vi "ReadAODVolume.vi"(8 "error in":errorcluster, 11 "FilePath":path) -> (0 "error out":errorcluster, 3 "settings_um":dbl[][](array[numeric]))   [LabVIEW 2014]
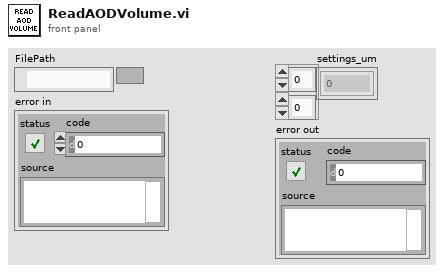
[diagram p1: front panel]
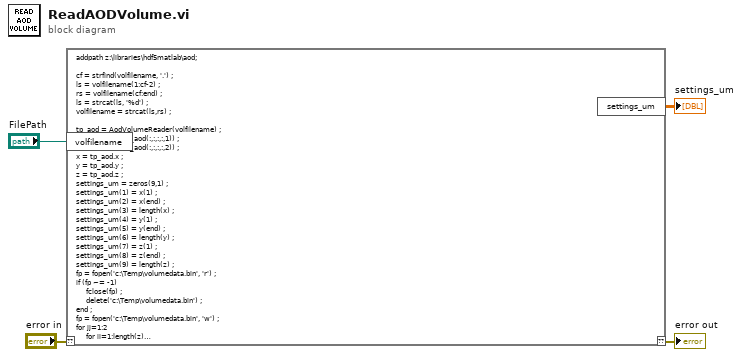
[diagram p0: block diagram]
diagram:
  n1 = script code="addpath z:\\libraries\\hdf5matlab\\aod;\n\ncf = strfind(volfilename, '.') ;\nls = volfilename(1:cf-2) ;\nrs = volfilename(cf:end) ;\nls = strcat(ls, '%d') ;\nvolfilename = strcat(ls,rs) ;\n\ntp_aod = AodVolumeReader(volfilename) ;\nvc1 = double(tp_aod(:,:,:,:,1)) ;\nvc2 = double(tp_aod(:,:,:,:,2)) ;\nx = tp_aod.x ;\ny = tp_aod.y ;\nz = tp_aod.z ;\nsettings_um = zeros(9,1) ;\nsettings_um(1) = x(1) ;\nsettings_um(2) = x(end) ;\nsettings_um(3) = length(x) ;\nsettings_um(4) = y(1) ;\nsettings_um(5) = y(end) ;\nsettings_um(6) = length(y) ;\nsettings_um(7) = z(1) ;\nsettings_um(8) = z(end) ;\nsettings_um(9) = length(z) ;\nfp = fopen('c:\\Temp\\volumedata.bin', 'r') ;\nif (fp ~= -1)\n     fclose(fp) ;\n     delete('c:\\Temp\\volumedata.bin') ;\nend ;\nfp = fopen('c:\\Temp\\volumedata.bin', 'w') ;\nfor jj=1:2\n     for ii=1:length(z)\n          if (jj==1)\n             tvol = vc1(:,:,ii) ; % write each frame in row order\n          else\n             tvol = vc2(:,:,ii) ;\n          end ;\n          fwrite(fp, tvol, 'int32') ;\n     end ;\nend ;\nfclose(fp) ;\nclearvars vc1 vc2 tvol"("??"="error in", "volfilename"="FilePath") -> ("??"=→"error out":errorcluster, "settings_um"=→"settings_um":dbl[][])
